vi "CalculateDestiny.vi"(8 "error in (no error)":errorcluster, 11 "AlignSkill in":refnum<class "AlignSkill.lvclass">) -> (0 "error out":errorcluster, 3 "AlignSkill out":refnum<class "AlignSkill.lvclass">)   [LabVIEW 2023, in "AlignSkill.lvclass"]
uses:
  AlignSkill.lvclass
  C:/Users/ebert/Documents/codes/SSL/repo/SSL_AI/GoToSkill_class/GoToSkill.lvclass
  <vilib>/Analysis/_algsub.llb/Real Vector Norm.vi
  <vilib>/Analysis/NI_AALPro.lvlib
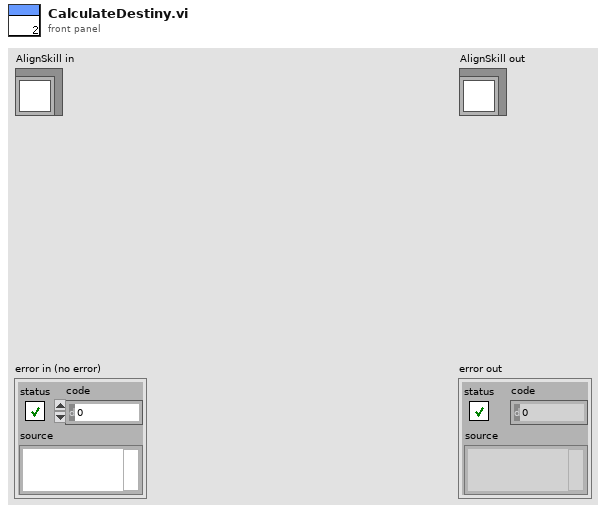
[diagram p1: front panel]
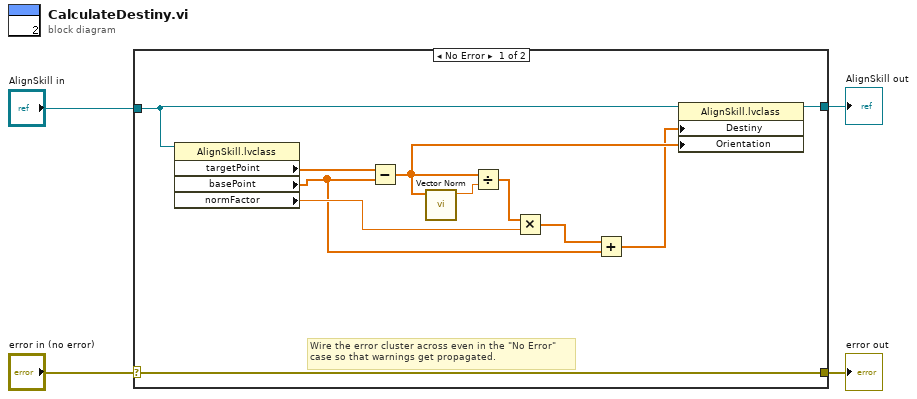
[diagram p0: block diagram]
diagram:
  n1 = case shown="No Error" "error in (no error)" {
    selector: "error in (no error)" -> [w15 w17]
    tunnel: [w15 w17] -> w3
    tunnel: [w7 w16] -> w1
    tunnel: "AlignSkill in" -> [w8 w16]
    frame No Error {
      # "Wire the error cluster across even in the \"No Error\"\ncase so that warnings get propagated."
      n2 = property class="AlignSkill.lvclass"(reference=w8) -> ("targetPoint"=w14:dbl[], "basePoint"=w10:dbl[], "normFactor"=w11:dbl)  [unwired: 1 in, 2 out]
      n3 = Subtract(x=w14, y=w10) -> (x-y=w6:dbl[])
      n4 = call-poly <vilib>:"Vector Norm.vi"("Input Vector"=w6) -> ("norm"=w13:dbl)  [unwired: 9 in, 1 out]
      n5 = Divide(x=w6, y=w13) -> (x/y=w12:dbl[])
      n6 = Multiply(x=w12, y=w11) -> (x*y=w9:dbl[])
      n7 = Add(x=w9, y=w10) -> (x+y=w5:dbl[])
      n8 = property class="AlignSkill.lvclass"(reference=w8, "Destiny"=w5, "Orientation"=w6) -> (reference out=w7:refnum<class "AlignSkill.lvclass">)  [unwired: 1 in, 1 out]
    }
    frame Error {
    }
  }
  "error out" <- w3
  "AlignSkill out" <- w1
